vi "New Message.vi"(6 "Receiving Actor":refnum<class "Message Enqueuer.lvclass">, 8 "error in (no error)":errorcluster, 9 "Message":refnum<class "Message.lvclass">, 10 "Time Stamp":timestamp, 11 "Message Logger in":refnum<class "Classic Logger.lvclass">) -> (0 "error out":errorcluster, 3 "Message Logger out":refnum<class "Classic Logger.lvclass">)   [LabVIEW 2020, in "Monitored Actor.lvlib" / "Classic Logger.lvclass"]
doc: "Called any time a monitored actor receives a message\n\nCopyright: MGI 2016\nAuthor: Derek Trepanier"
uses:
  <vilib>/MGI/Monitored Actor/Classic Monitor/Logger/Classic Logger Actor/Classic Logger.lvclass
  <vilib>/ActorFramework/Message/Message.lvclass
  <vilib>/ActorFramework/Message Enqueuer/Message Enqueuer.lvclass
  <vilib>/MGI/Monitored Actor/Classic Monitor/Logger/Classic Logger Actor/Monitor Data.ctl
  <vilib>/MGI/Monitored Actor/Classic Monitor/Logger/Classic Logger Actor/Classic Logger.lvclass/Classic Logger.ctl
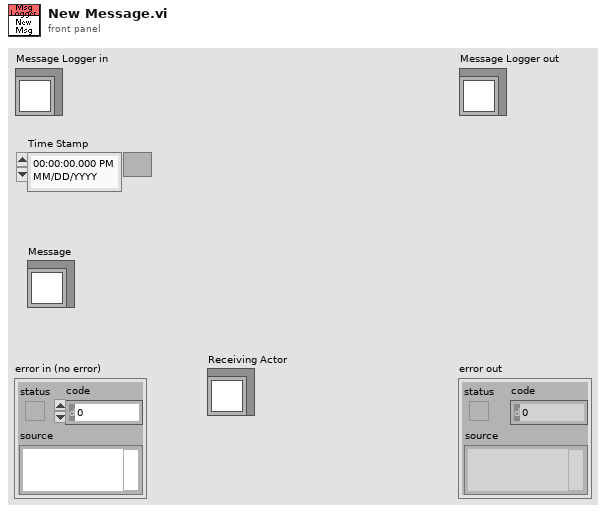
[diagram p1: front panel]
types:
  T1 = typedef "Monitored Actor.lvlib/Classic Logger.lvclass/Monitor Data.ctl" = cluster{"Time Stamp":timestamp, "class name":string, "Msg XML":string}
  T2 = cluster{"Time Stamp":timestamp, "class name":string, "xml string":string}
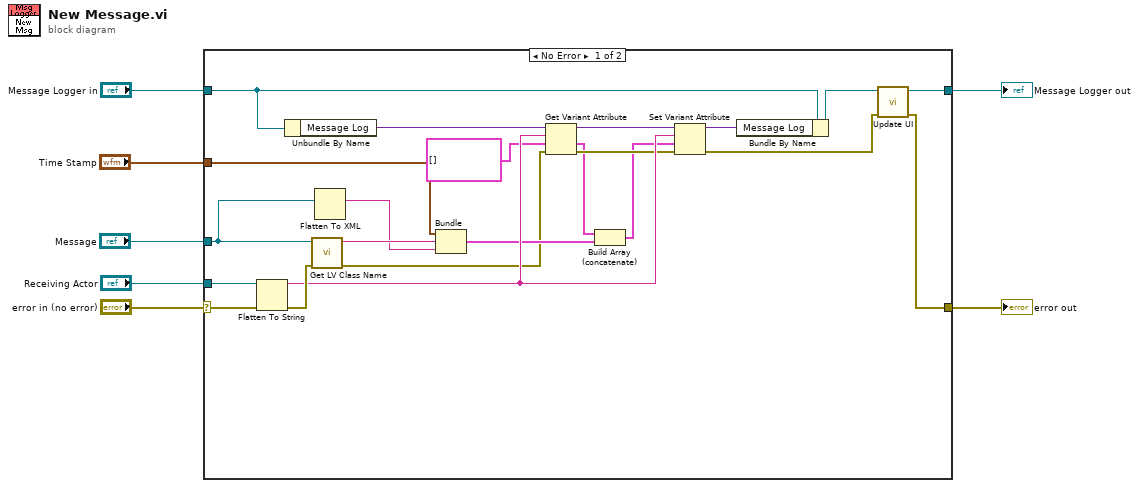
[diagram p0: block diagram]
diagram:
  n1 = case shown="No Error" "error in (no error)" {
    selector: "error in (no error)" -> [w24 w30]
    tunnel: [w10 w30] -> w7
    tunnel: [w12 w31] -> w6
    tunnel: "Receiving Actor" -> [w28 _]
    tunnel: "Message" -> [w9 _]
    tunnel: "Time Stamp" -> [w27 _]
    tunnel: "Message Logger in" -> [w29 w31]
    frame No Error {
      n2 = Flatten To String(anything=w28, error in (no error)=w24) -> (data string=w21:string, error out=w25:errorcluster)  [unwired: 2 in, 1 out]
      n3 = Unbundle By Name(w29) -> ("Message Log"=w22:variant)
      n4 = call <vilib>:"Get LV Class Name.vi"("error in (no error)"=w25, "object"=w9) -> ("error out"=w15:errorcluster, "class name"=w26:string)  [unwired: 8 in]
      n5 = Flatten To XML(6:w9) -> (2:w8:string)
      n6 = Bundle("Time Stamp"=w27, "class name"=w26, "xml string"=w8) -> (w17:T2)  [unwired: 1 in]
      n7 = Get Variant Attribute(Variant=w22, name=w21, default value (empty Variant)=T1[] [], error in=w15) -> (duplicate Variant=w23:variant, value=w18:T1[], error out=w19:errorcluster)  [unwired: 1 out]
      n8 = Build Array (concatenate)(w18, w17) -> (w16:T1[])
      n9 = Set Variant Attribute(Variant=w23, name=w21, value=w16, error in=w19) -> (Variant out=w14:variant, error out=w11:errorcluster)  [unwired: 1 out]
      n10 = Bundle By Name(cluster=w29, "Message Log"=w14) -> (w13:refnum<class "Classic Logger.lvclass">)
      n11 = call <vilib>:"Update UI.vi"("error in (no error)"=w11, "Message Logger in"=w13) -> ("error out"=w10:errorcluster, "Message Logger out"=w12:refnum<class "Classic Logger.lvclass">)  [unwired: 8 in]
    }
    frame Error {
    }
  }
  "error out" <- w7
  "Message Logger out" <- w6
